vi "Normal Step 1 (SubVI).vi"(0 "aLC":dbl, 5 "aRC":dbl, 7 "Ldist":dbl, 9 "Rdist":dbl, 11 "Rside":dbl) -> (4 "lbrc":dbl, 6 "rblc":dbl, 8 "aLB2":dbl, 10 "aRB2":dbl)   [LabVIEW 2015]
uses:
  <vilib>/express/express arith-compare/Formula/XNode/ExpressFormulaBlockNode.xnode
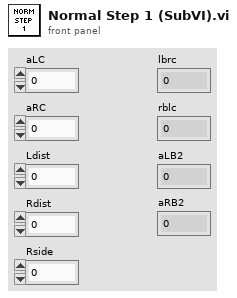
[diagram p1: front panel]
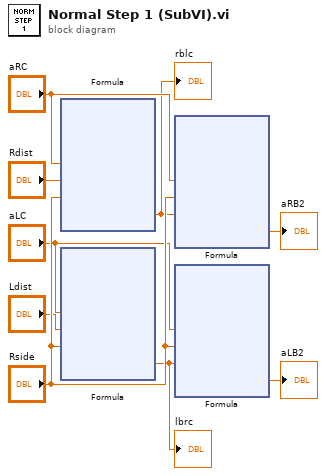
[diagram p0: block diagram]
diagram:
  n1 = xnode "Formula"("aRC"="aRC", "Rdist"="Rdist", "Rside"="Rside") -> ("Result"=w7:dbl)  [unwired: 1 in, 1 out]
  "rblc" <- w7
  n2 = xnode "Formula"("aLC"="aLC", "Ldist"="Ldist", "Rside"="Rside") -> ("Result"=w3:dbl)  [unwired: 1 in, 1 out]
  "lbrc" <- w3
  n3 = xnode "Formula"("aRC"="aRC", "RSide"="Rside", "rblc"=w7) -> ("Result"=→"aRB2":dbl)  [unwired: 1 in, 1 out]
  n4 = xnode "Formula"("aLC"="aLC", "Rside"="Rside", "lbrc"=w3) -> ("Result"=→"aLB2":dbl)  [unwired: 1 in, 1 out]
